vi "CCD_PDA_ErrorHandler.vi"(6 "error in":errorcluster) -> (0 "error out":errorcluster, 3 "All-Quit":bool)   [LabVIEW 2019]
doc: "Resets the CCD camera controller and initializes it with Setup String. The default Setup String is \"ldb,1,16,u,0,225,25,b,1,15;sdu,0,1024,1024;cl0;omrm;sron\". \nError, if no -1, is set as 0 if a serial poll detects an error (bit 15 in status bit set)\n\nSet the CCD Setup String Global variable after the command is complete."
uses:
  <vilib>/Utility/error.llb/DialogType.ctl
  Globals and TypeDefs/Type Definitions.llb/3 way Status.ctl
  Globals and TypeDefs/gDetector.vi
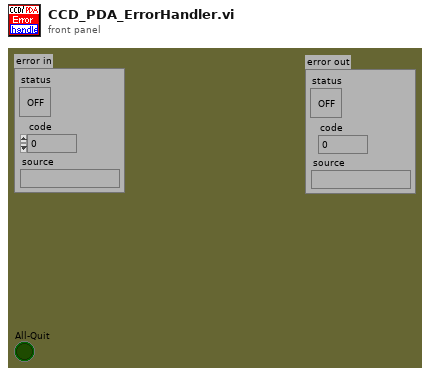
[diagram p1: front panel]
types:
  T1 = enum16{"--Quit--", "Init GPIB", "Poll GPIB", "Wait for SRQ", "Clear CCD Parameters", "New CCD Parameters", "Check CCD Command Error"}
  T2 = enum16{"End", "Init", "Reset", "SetAcqParameter", "SetArea", "Start Acquisition", "Busy Status Poll", "Read", "Stop"}
  T3 = typedef "DialogType.ctl" = u16
  T4 = typedef "Error Categories.ctt" = enum8{"General", "CCD-256x1024", "CCD-1340x400", "InGaAs PDA", "McPherson 2075", "Magnetic Field", "Temperature Control", "Other"}
  T5 = enum16{"Left Button", "Center Button", "Right Button", "Window Close"}
  T6 = typedef "3 way Status.ctl" = u8
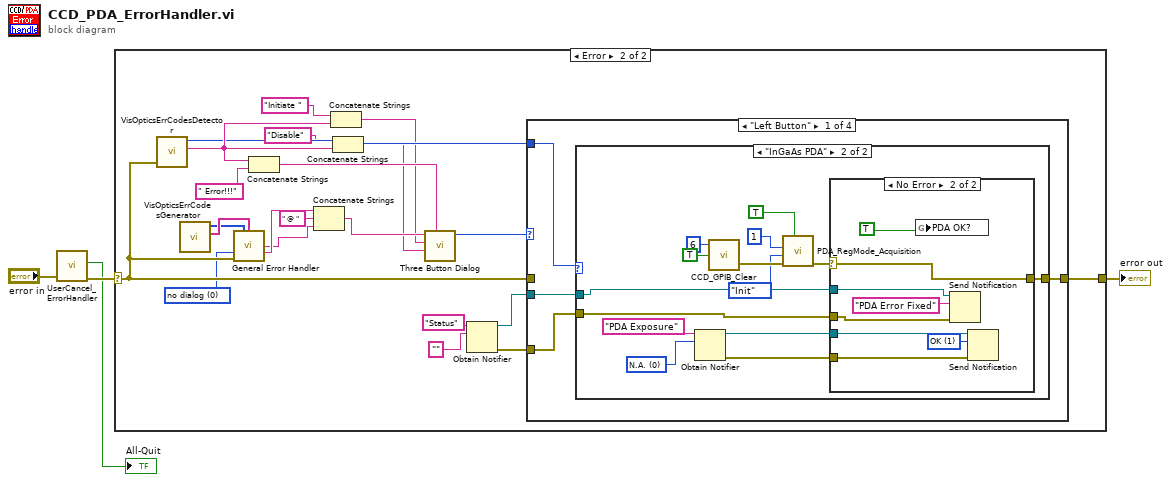
[diagram p0: block diagram]
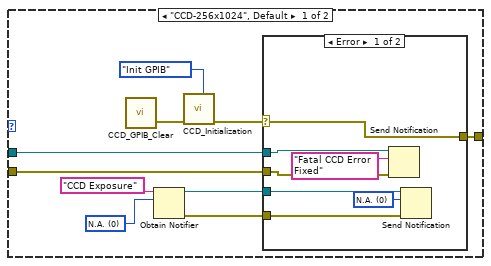
[diagram p3: hidden frame]
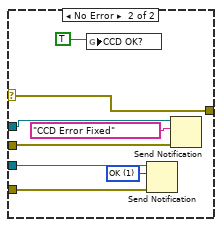
[diagram p4: hidden frame]
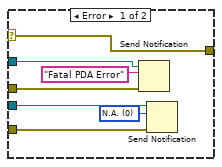
[diagram p5: hidden frame]
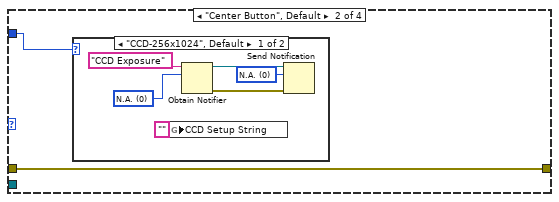
[diagram p6: hidden frame]
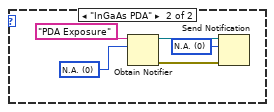
[diagram p7: hidden frame]
diagram:
  n1 = call "UserCancel_ErrorHandler.vi"("error in"="error in") -> ("error out"=w2:errorcluster, "All-Quit"=→"All-Quit":bool)  [unwired: 5 in, 1 out]
  n2 = case shown="Error" w2 {
    selector: w2 -> [w5 w26]
    tunnel: [w5 w27] -> w4
    frame No Error {
    }
    frame Error {
      w21 = T3 0 items=["no dialog", "OK message", "continue or stop message", "OK message + warnings", "continue/stop + warnings"] ("type of dialog (OK msg:1)")
      n3 = call "VisOpticsErrCodesDetector.vi"("error in"=w26) -> ("NHMFL Visible Optics Error Category"=w24:T4, "Error Category text"=w25:string)  [unwired: 2 in, 2 out]
      n4 = call "VisOpticsErrCodesGenerator.vi"() -> ("user-defined descriptions"=w23:string[], "user-defined codes"=w22:i32[])  [unwired: 3 in, 4 out]
      n5 = call <vilib>:"General Error Handler.vi"("[user-defined codes]"=w22, "[user-defined descriptions]"=w23, "type of dialog (OK msg:1)"=w21, "error in (no error)"=w26) -> ("source out"=w15:string, "message"=w17:string)  [unwired: 7 in, 3 out]
      n6 = Concatenate Strings(w25, " Error!!!" ("string")) -> (w18:string)
      n7 = Concatenate Strings(w17, " @ " ("string"), w15) -> (w14:string)
      n8 = Concatenate Strings("Initiate " ("Left Button Text (\"Yes\")"), w25) -> (w12:string)
      n9 = Concatenate Strings("Disable" ("Center Button Text (\"No\")"), w25) -> (w10:string)
      n10 = call <vilib>:"Three Button Dialog.vi"("Window Title (\"\")"=w18, "Center Button Text (\"No\")"=w10, "Left Button Text (\"Yes\")"=w12, "message"=w14) -> ("Which Button?"=w20:T5)  [unwired: 7 in]
      n11 = Obtain Notifier(name (unnamed)="Status", notification data type="" ("Status")) -> (notifier out=w7:refnum<notifier>, error out=w6:errorcluster)  [unwired: 2 in, 1 out]
      n12 = case shown="\"Left Button\"" w20 {
        tunnel: [w31 w87 w99 w100] -> w27
        tunnel: w26 -> [_ w87 w99 w100]
        tunnel: w24 -> [w30 w86 _ _]
        tunnel: w7 -> [w29 _ _ _]
        tunnel: w6 -> [w28 _ _ _]
        frame "Left Button" {
          n13 = case shown="\"InGaAs PDA\"" w30 {
            tunnel: [w38 w68] -> w31
            tunnel: w29 -> [w33 w58]
            tunnel: w28 -> [w32 w57]
            frame "CCD-256x1024", Default {
              w37 = T6 0 items=["N.A.", "OK", "Busy", "Done"] ("H(T)")
              n14 = call "CCD_GPIB_Clear.vi"() -> ("error out"=w40:errorcluster)  [unwired: 5 in]
              n15 = Obtain Notifier(name (unnamed)="CCD Exposure", notification data type=w37) -> (notifier out=w35:refnum<notifier>, error out=w34:errorcluster)  [unwired: 2 in, 1 out]
              n16 = call "CCD_Initialization.vi"("error in"=w40, "Starting Action"=T1."Init GPIB") -> ("error out"=w39:errorcluster)  [unwired: 3 in, 4 out]
              n17 = case shown="Error" w39 {
                selector: w39 -> [w45 w52]
                tunnel: w35 -> [w47 w54]
                tunnel: w34 -> [w46 w53]
                tunnel: [w45 w52] -> w38
                tunnel: w33 -> [w43 w50]
                tunnel: w32 -> [w42 w49]
                frame Error {
                  w48 = T6 0 items=["N.A.", "OK", "Busy", "Done"] ("notification")
                  n18 = Send Notification(notification="Fatal CCD Error Fixed", notifier=w43, error in (no error)=w42) -> ()  [unwired: 2 out]
                  n19 = Send Notification(notification=w48, notifier=w47, error in (no error)=w46) -> ()  [unwired: 2 out]
                }
                frame No Error {
                  w56 = T6 1 items=["N.A.", "OK", "Busy", "Done"] ("notification")
                  n20 = global write "gDetector.vi" "CCD OK?"(TRUE ("CCD OK?")) -> ()
                  n21 = Send Notification(notification=w56, notifier=w54, error in (no error)=w53) -> ()  [unwired: 2 out]
                  n22 = Send Notification(notification="CCD Error Fixed", notifier=w50, error in (no error)=w49) -> ()  [unwired: 2 out]
                }
              }
            }
            frame "InGaAs PDA" {
              w62 = T6 0 items=["N.A.", "OK", "Busy", "Done"] ("H(T)")
              n23 = Obtain Notifier(name (unnamed)="PDA Exposure", notification data type=w62) -> (notifier out=w60:refnum<notifier>, error out=w59:errorcluster)  [unwired: 2 in, 1 out]
              n24 = call "CCD_GPIB_Clear.vi"("Device Clear?"=TRUE, "GPIB Address"=i16 6) -> ("error out"=w70:errorcluster)  [unwired: 3 in]
              n25 = call "PDA_RegMode_Acquisition.vi"("Shutter"=TRUE, "error in"=w70, "StartIng Mode"=T2."Init", "Number of Cycles"=u32 1) -> ("error out"=w69:errorcluster)  [unwired: 1 in, 3 out]
              n26 = case shown="No Error" w69 {
                selector: w69 -> [w74 w81]
                tunnel: w60 -> [w76 w83]
                tunnel: w59 -> [w75 w82]
                tunnel: [w74 w81] -> w68
                tunnel: w58 -> [w72 w79]
                tunnel: w57 -> [w71 w78]
                frame Error {
                  w77 = T6 0 items=["N.A.", "OK", "Busy", "Done"] ("notification")
                  n27 = Send Notification(notification="Fatal PDA Error", notifier=w72, error in (no error)=w71) -> ()  [unwired: 2 out]
                  n28 = Send Notification(notification=w77, notifier=w76, error in (no error)=w75) -> ()  [unwired: 2 out]
                }
                frame No Error {
                  w85 = T6 1 items=["N.A.", "OK", "Busy", "Done"] ("notification")
                  n29 = global write "gDetector.vi" "PDA OK?"(TRUE ("CCD OK?")) -> ()
                  n30 = Send Notification(notification="PDA Error Fixed", notifier=w79, error in (no error)=w78) -> ()  [unwired: 2 out]
                  n31 = Send Notification(notification=w85, notifier=w83, error in (no error)=w82) -> ()  [unwired: 2 out]
                }
              }
            }
          }
        }
        frame "Center Button", Default {
          n32 = case shown="\"CCD-256x1024\", Default" w86 {
            frame "CCD-256x1024", Default {
              w89 = T6 0 items=["N.A.", "OK", "Busy", "Done"] ("notification")
              w93 = T6 0 items=["N.A.", "OK", "Busy", "Done"] ("H(T)")
              n33 = global write "gDetector.vi" "CCD Setup String"("" ("CCD Setup String")) -> ()
              n34 = Obtain Notifier(name (unnamed)="CCD Exposure", notification data type=w93) -> (notifier out=w91:refnum<notifier>, error out=w90:errorcluster)  [unwired: 2 in, 1 out]
              n35 = Send Notification(notification=w89, notifier=w91, error in (no error)=w90) -> ()  [unwired: 2 out]
            }
            frame "InGaAs PDA" {
              w94 = T6 0 items=["N.A.", "OK", "Busy", "Done"] ("notification")
              w98 = T6 0 items=["N.A.", "OK", "Busy", "Done"] ("H(T)")
              n36 = Obtain Notifier(name (unnamed)="PDA Exposure", notification data type=w98) -> (notifier out=w96:refnum<notifier>, error out=w95:errorcluster)  [unwired: 2 in, 1 out]
              n37 = Send Notification(notification=w94, notifier=w96, error in (no error)=w95) -> ()  [unwired: 2 out]
            }
          }
        }
        frame "Right Button" {
        }
        frame "Window Close" {
        }
      }
    }
  }
  "error out" <- w4
